vi "Push block to shooter.vi"(8 "error in (no error)":errorcluster, 10 "Shoot?":bool) -> (0 "error out":errorcluster)   [LabVIEW 2017]
uses:
  <vilib>/Rock Robotics/WPI/Solenoid/WPI_SolenoidValue.ctl
  <vilib>/Rock Robotics/WPI/Solenoid/WPI_SolenoidSetEnum.vi
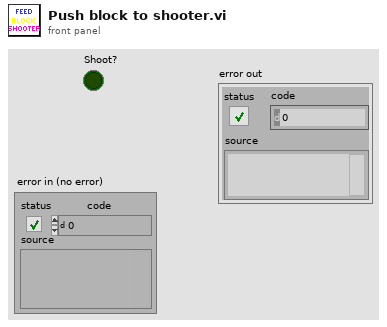
[diagram p1: front panel]
types:
  T1 = typedef "WPI_SolenoidDevRef.ctl" = cluster{"DevStatus":errorcluster, "Pneumatics Control Module":u8, "Forward Solenoid Channel":T2, "Reverse Solenoid Channel":T2}
  T2 = typedef "WPI_SolenoidChannel.ctl" = enum8{"Solenoid 0", "Solenoid 1", "Solenoid 2", "Solenoid 3", "Solenoid 4", "Solenoid 5", "Solenoid 6", "Solenoid 7", "Invalid"}
  T3 = typedef "WPI_SolenoidValue.ctl" = enum16{"Off", "On", "Forward", "Reverse"}
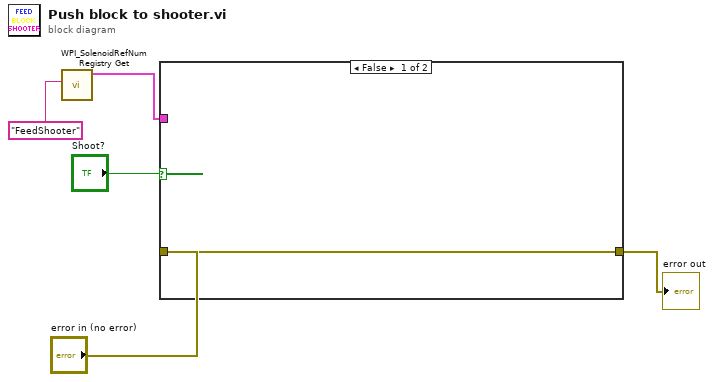
[diagram p0: block diagram]
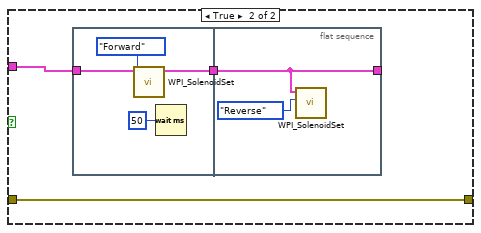
[diagram p2: hidden frame]
diagram:
  n1 = call <vilib>:"WPI_SolenoidRefNum Registry Get.vi"("refnum name"="FeedShooter") -> ("SolenoidDevRef"=w1:T1)  [unwired: 9 in, 1 out]
  n2 = case shown="False" "Shoot?" {
    tunnel: "error in (no error)" -> [w6 w9]
    tunnel: [w6 w9] -> w5
    tunnel: w1 -> [_ w8]
    frame False {
    }
    frame True {
      n3 = flat-sequence {
        tunnel: w8 -> [w11]
        tunnel: [w12] -> w7
        tunnel: [w14] -> _
        tunnel: w7 -> [w14]
        frame #0 {
          n4 = call-poly <vilib>:"WPI_SolenoidSet.vi"("Value"=WPI_SolenoidValue."Forward", "SolenoidDevRef"=w11) -> ("SolenoidDevRef"=w12:T1)  [unwired: 8 in, 1 out]
          n5 = Wait (ms)(milliseconds to wait=u32 50) -> ()  [unwired: 1 out]
        }
        frame #1 {
          n6 = call-poly <vilib>:"WPI_SolenoidSet.vi"("Value"=WPI_SolenoidValue."Reverse", "SolenoidDevRef"=w14) -> ()  [unwired: 8 in, 2 out]
        }
      }
    }
  }
  "error out" <- w5
